vi "Sum 2D [xo] (DBL).vi"(1 "2D":dbl[][](array[numeric])) -> (0 "1D":dbl[](array[numeric]))   [LabVIEW 2009]
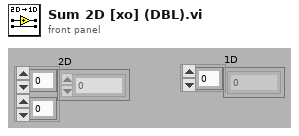
[diagram p1: front panel]
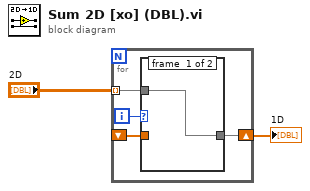
[diagram p0: block diagram]
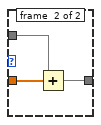
[diagram p2: hidden frame]
diagram:
  n1 = for {
    tunnel: "2D" -> [w4] mode=indexing
    shift-right: [w5] -> w1
    shift-left: _ -> [w3]
    i -> [w6]
    n2 = case shown="1, Default" w6 {
      tunnel: [w7 w10] -> w5
      tunnel: w4 -> [w7 w9]
      tunnel: w3 -> [_ w8]
      frame #0 {
      }
      frame #1 {
        n3 = Add(x=w9, y=w8) -> (x+y=w10:dbl[])
      }
    }
  }
  "1D" <- w1
